vi "ColseAC230V_L.vi"(0 "datain":string[](array[string])=["备注", "负载通道", "负载地址", "延时时间", "output max", "output min", "量测类型", "待测物板号"], 5 "HW CH Number":i32, 7 "Setup":string) -> (4 "REPORT INDECATE":string[][](array[string])=[["微安测试", "", "", "", ""], ["微安量测", "4", "0.000", "0.1", "NG"], ["微安量测", "4", "0.000", "0.1", "NG"], ["微安量测", "4", "0.000", "0.1", "NG"], ["微安量测", "4", "0.000", "0.1", "NG"]], 6 "ROW HEAD":string[](array[string]), 8 "PF":string[](array[string]), 10 "testData":string[](array[string]), 15 "Array":string[](array[string]))   [LabVIEW 2018]
uses:
  Subvi/Global.vi
panel:
  out "测试板数":i32
  out "数组":bool[](array[boolean])
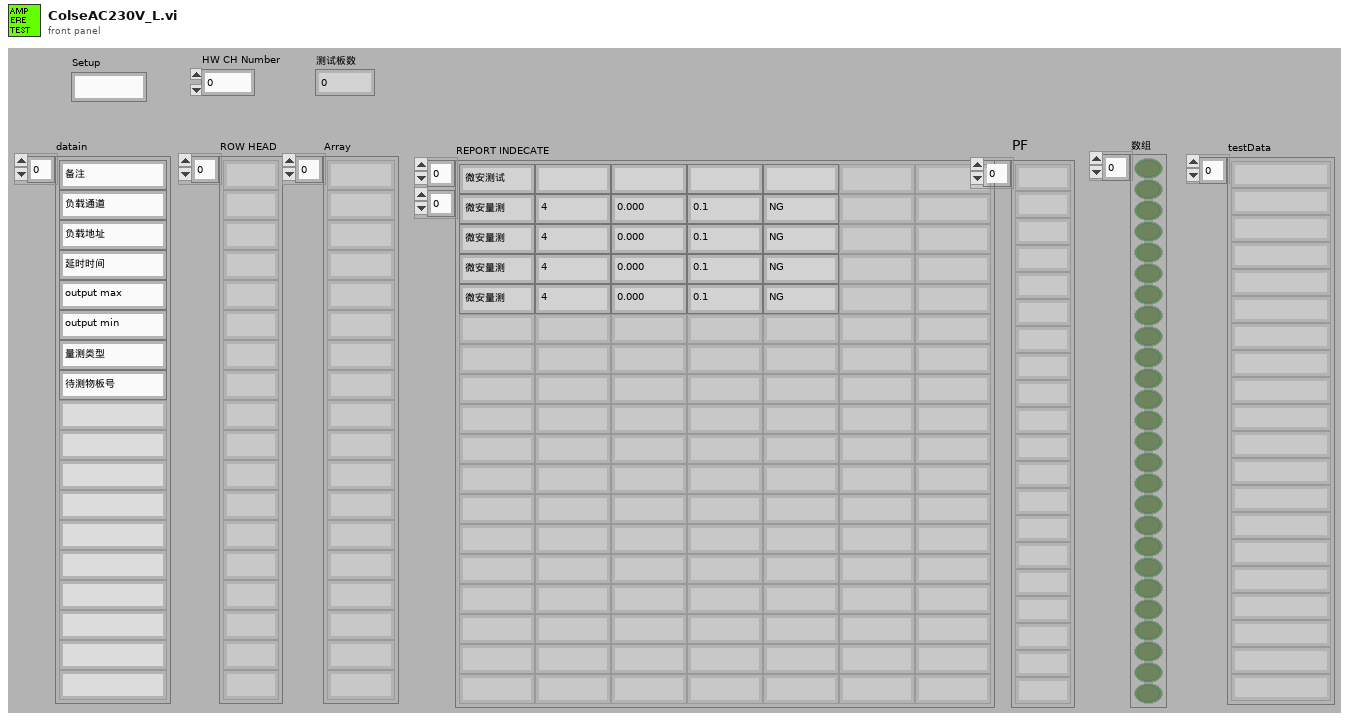
[diagram p1: front panel]
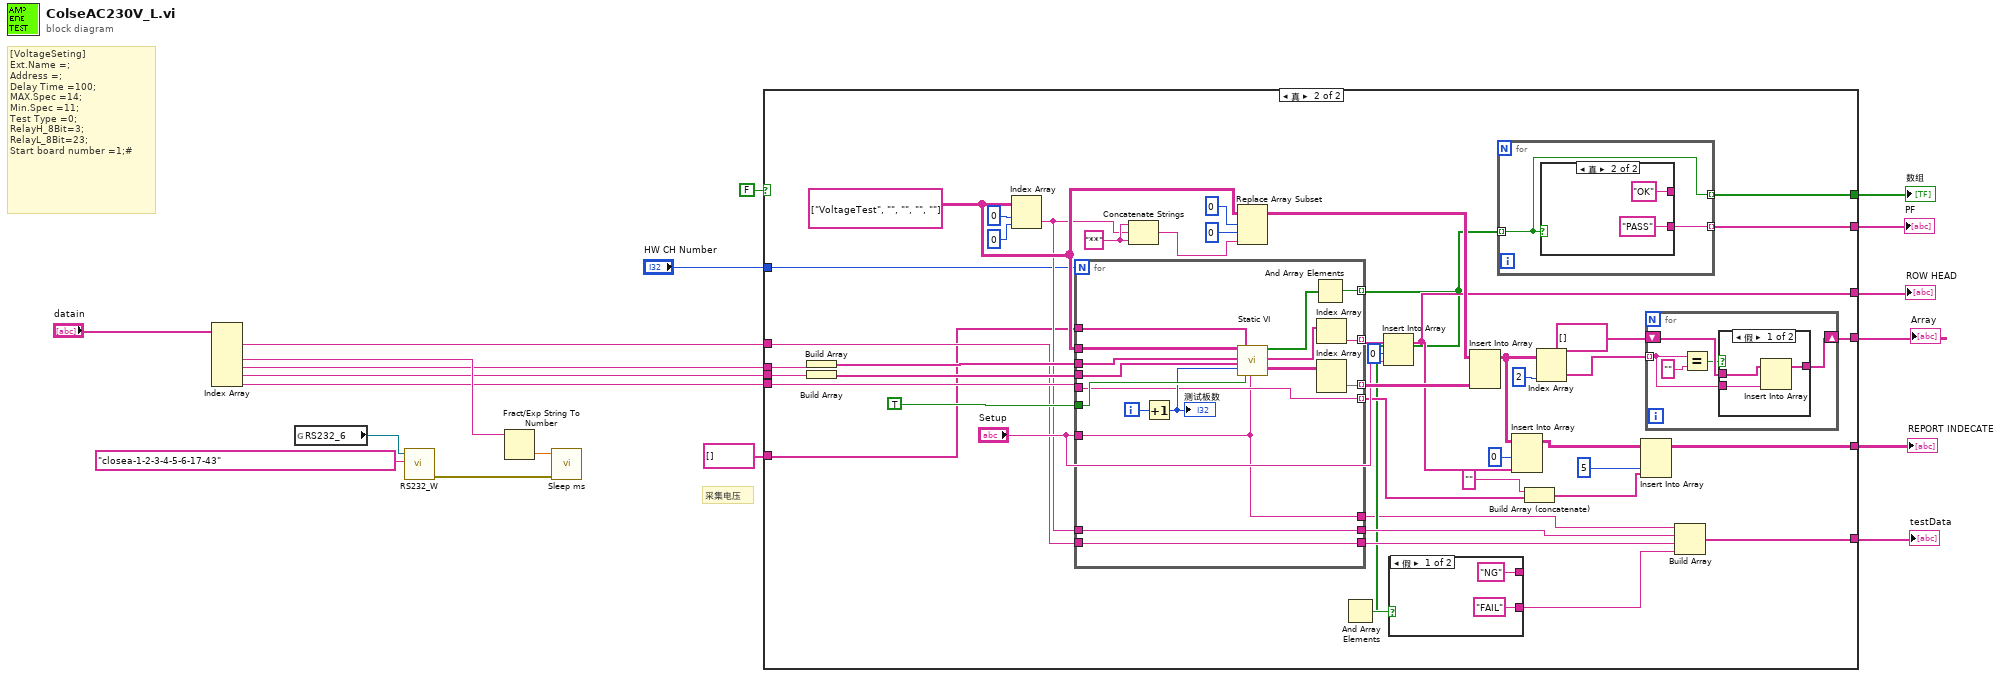
[diagram p0: block diagram]
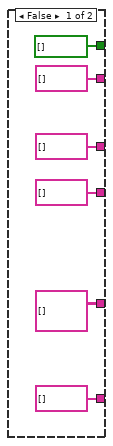
[diagram p2: hidden frame]
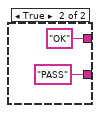
[diagram p3: hidden frame]
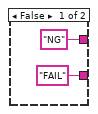
[diagram p4: hidden frame]
diagram:
  # "采集电压"
  # "[VoltageSeting]\nExt.Name =;\nAddress =;\nDelay Time =100;\nMAX.Spec =14;\nMin.Spec =11;\nTest Type =0;\nRelayH_8Bit=3;\nRelayL_8Bit=23;\nStart board number =1;#"
  n1 = Index Array(array="datain") -> (element #1=w10:string, element #3=w16:string, element #4=w15:string, element #5=w14:string, element #6=w12:string)  [unwired: 6 in, 1 out]
  n2 = global read "Global.vi" "RS232_6"() -> (w5:refnum<visa-resource-name>)
  n3 = call "RS232_W.vi"("CMD"="closea-1-2-3-4-5-6-17-43", "VISA资源名称"=w5) -> ("error out"=w1:errorcluster)  [unwired: 7 in, 2 out]
  n4 = Fract/Exp String To Number(string=w16) -> (number=w6:dbl)  [unwired: 3 in, 1 out]
  n5 = call "Sleep ms.vi"("error in (no error)"=w1, "等待时间（毫秒）"=w6) -> ()  [unwired: 9 in, 1 out]
  n6 = case shown="真" FALSE {
    tunnel: [string[] [] ("Array") w66] -> w19
    tunnel: [string[] [] w65] -> w18
    tunnel: w15 -> [_ w58]
    tunnel: w14 -> [_ w57]
    tunnel: [string[] [] w46] -> w13
    tunnel: w12 -> [_ w44]
    tunnel: [string[][] [] w41] -> w11
    tunnel: w10 -> [_ w36]
    tunnel: [string[] [] w30] -> w9
    tunnel: [bool[] [] w28] -> w8
    tunnel: "HW CH Number" -> [_ w27]
    tunnel: string[] [] ("Out data") -> [_ w26]
    frame False {
    }
    frame True {
      w56 = string[][] [["VoltageTest", "", "", "", ""]]
      w62 = "**" ("字符串")
      n7 = Build Array(w58) -> (w55:string[])
      n8 = Build Array(w57) -> (w54:string[])
      n9 = Index Array(array=w56, index (row)=0 ("索引 (行)"), index (col)=0 ("禁用的索引 (列)")) -> (element=w37:string)
      n10 = for {
        N: w27 -> [_]
        tunnel: w26 -> [w90]
        tunnel: w55 -> [w88]
        tunnel: w54 -> [w87]
        tunnel: "Setup" -> [w74]
        tunnel: TRUE -> [w85]
        tunnel: [w83] -> w32 mode=indexing
        tunnel: [w80] -> w50 mode=indexing
        tunnel: w56 -> [w89]
        tunnel: [w78] -> w51 mode=indexing
        tunnel: w44 -> [w77]
        tunnel: [w77] -> w40 mode=indexing
        tunnel: w37 -> [w76]
        tunnel: [w76] -> w35
        tunnel: w36 -> [w75]
        tunnel: [w75] -> w34
        tunnel: [w74] -> w29
        i -> [w82]
        n11 = Increment(x=w82) -> (x+1=w84:i32)
        "测试板数" <- w84
        n12 = call "Static VI.vi"("添加的数组"=w89, "Max"=w88, "Min"=w87, "板数"=w84, "INPUTSTRING"=w90, "是否为字符串对比"=w85, "SQ"=w74) -> ("P/F"=w86:bool[], "SQ out"=w81:string[], "arrauy out"=w79:string[][])  [unwired: 9 in, 1 out]
        n13 = And Array Elements(Boolean array=w86) -> (logical AND=w83:bool)
        n14 = Index Array(array=w81) -> (element=w80:string)  [unwired: 1 in]
        n15 = Index Array(array=w79) -> (element=w78:string[])  [unwired: 2 in]
      }
      n16 = Concatenate Strings(w62, w37, w62) -> (w59:string)
      n17 = Replace Array Subset(array=w56, new element=w59, index (row)=0 ("索引 (行)"), index (col)=0 ("禁用的索引 (列)")) -> (w52:string[][])
      n18 = And Array Elements(Boolean array=w32) -> (logical AND=w33:bool)
      n19 = Insert Into Array(array=w50, index=0 ("索引"), new element="Setup") -> (w46:string[])
      n20 = case shown="假" w33 {
        tunnel: ["NG" "OK"] -> _
        tunnel: ["FAIL" "PASS"] -> w31
        frame False {
        }
        frame True {
        }
      }
      n21 = Insert Into Array ("数组插入")(array=w52, new element=w51) -> (w47:string[][])  [unwired: 2 in]
      n22 = for {
        tunnel: w32 -> [w91] mode=indexing
        tunnel: [w92] -> w65 mode=indexing
        tunnel: [w91] -> w28 mode=indexing
        n23 = case shown="真" w91 {
          tunnel: ["NG" "OK"] -> _
          tunnel: ["FAIL" "PASS"] -> w92
          frame False {
          }
          frame True {
          }
        }
      }
      n24 = Insert Into Array(array=w47, index (col)=0 ("禁用的索引 (列)"), new element=w46) -> (w42:string[][])  [unwired: 1 in]
      n25 = Build Array (concatenate)("" ("字符串"), w40) -> (w38:string[])
      n26 = Index Array(array=w47, index (col)=2 ("禁用的索引 (列)")) -> (element=w67:string[])  [unwired: 1 in]
      n27 = Insert Into Array(array=w42, index (col)=5 ("禁用的索引 (列)"), new element=w38) -> (w41:string[][])  [unwired: 1 in]
      n28 = for {
        tunnel: w67 -> [w97] mode=indexing
        shift-right: [w98] -> w66
        shift-left: string[] [] ("Array") -> [w101]
        n29 = Equal?(x=w97, y="") -> (x = y?=w99:bool)
        n30 = case shown="假" w99 {
          tunnel: w101 -> [w104 w105]
          tunnel: [w103 w105] -> w98
          tunnel: w97 -> [w102 _]
          frame False {
            n31 = Insert Into Array(array=w104, new element=w102) -> (w103:string[])  [unwired: 1 in]
          }
          frame True {
          }
        }
      }
      n32 = Build Array(w29, w35, w34, w31) -> (w30:string[])
    }
  }
  "REPORT INDECATE" <- w11
  "ROW HEAD" <- w13
  "PF" <- w18
  "Array" <- w19
  "数组" <- w8
  "testData" <- w9
